vi "UI Front Panel State.vi"(8 "error in (no error)":errorcluster, 9 "Front Panel Window:Behavior":T1(ring)=enum."Default", 10 "Argument":T2="Open", 11 "UI ActorTop in":refnum<class "UIActorTop2.lvclass">) -> (0 "error out":errorcluster, 3 "UI ActorTop out":refnum<class "UIActorTop2.lvclass">)   [LabVIEW 2021]
doc: "UI: Front Panel State\ninclude Open, close, standard, Hidden and FP.Center\n2015-03-18 16:41:03\n蒋松\njiangsong@outlook.com"
uses:
  <userlib>/sushu/Tools/Front Panel State.ctl
  UIActorTop2.lvclass
  <userlib>/sushu/sushu.lvlib
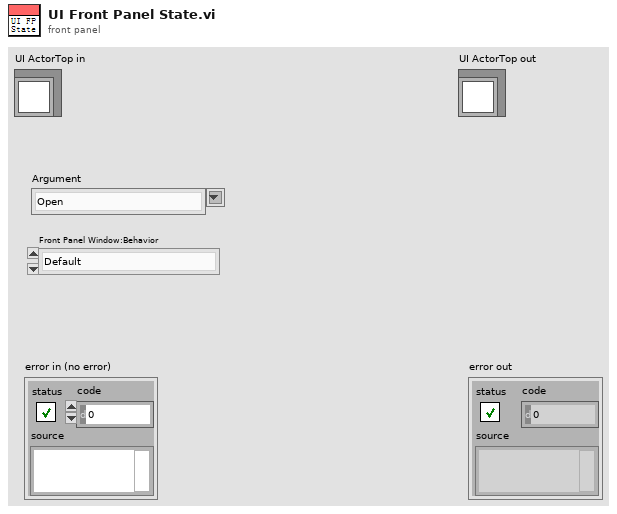
[diagram p1: front panel]
types:
  T1 = enum32{"Invalid", "Default", "Floating", "Floating/Auto-Hide", "Modal"}
  T2 = typedef "sushu.lvlib/Front Panel State.ctl" = string
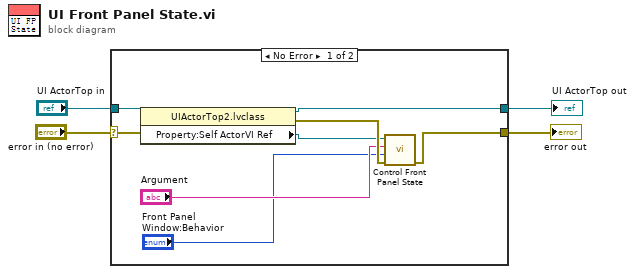
[diagram p0: block diagram]
diagram:
  n1 = case shown="No Error" "error in (no error)" {
    selector: "error in (no error)" -> [w11 w14]
    tunnel: [w10 w14] -> w3
    tunnel: [w9 w13] -> w1
    tunnel: "UI ActorTop in" -> [w12 w13]
    frame No Error {
      n2 = property class="UIActorTop2.lvclass"(reference=w12, error in=w11) -> (reference out=w9:refnum<class "UIActorTop2.lvclass">, error out=w8:errorcluster, "Property:Self ActorVI Ref"=w7:refnum<vi>)
      n3 = call <userlib>:"Control Front Panel State.vi"("error out"=w8, "Front Panel Window:Behavior"="Front Panel Window:Behavior", "Argument"="Argument", "Core.Current VI Reference"=w7) -> ("error out"=w10:errorcluster)  [unwired: 6 in, 1 out]
    }
    frame Error {
    }
  }
  "error out" <- w3
  "UI ActorTop out" <- w1
